vi "Load Font.vi"(11 "font directory":path) -> ()   [LabVIEW 2017]
uses:
  Default Settings.vi
panel:
  out "font overview":picture
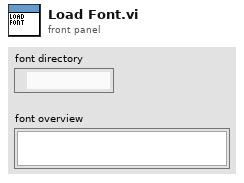
[diagram p1: front panel]
types:
  T1 = cluster{"left":i16, "top":i16, "right":i16, "bottom":i16}
  T2 = typedef "imagedata.ctl" = cluster{"image type":i32, "image depth":i32, "image":u8[], "mask":u8[], "colors":u32[], "Rectangle":cluster{"left":i16, "top":i16, "right":i16, "bottom":i16}}
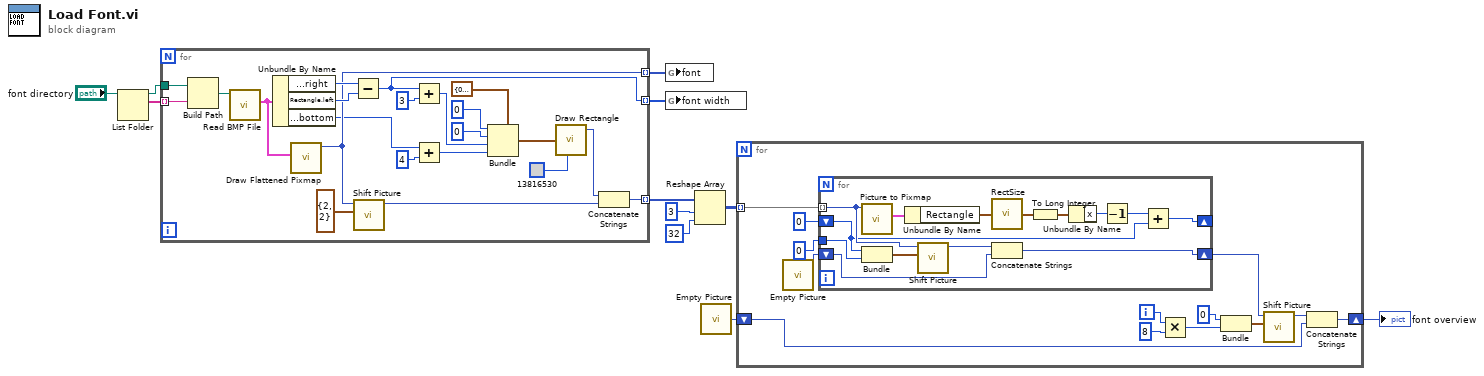
[diagram p0: block diagram]
diagram:
  n1 = List Folder(path="font directory") -> (path out=w11:path, filenames=w10:string[])  [unwired: 3 in, 2 out]
  n2 = for {
    tunnel: w10 -> [w32] mode=indexing
    tunnel: w11 -> [w33]
    tunnel: [w25] -> w8 mode=indexing
    tunnel: [w20] -> w7 mode=indexing
    tunnel: [w12] -> w6 mode=indexing
    n3 = Build Path(base path=w33, name or relative path=w32) -> (appended path=w31:path)
    n4 = call <vilib>:"Read BMP File.vi"("path to BMP file"=w31) -> ("image data"=w27:T2)  [unwired: 8 in, 2 out]
    n5 = Unbundle By Name(w27) -> ("Rectangle.right"=w30:i16, "Rectangle.left"=w29:i16, "Rectangle.bottom"=w17:i16)
    n6 = call <vilib>:"Draw Flattened Pixmap.vi"("image data"=w27) -> ("new picture"=w25:picture)  [unwired: 8 in]
    n7 = Subtract(x=w30, y=w29) -> (x-y=w20:i16)
    n8 = call "Shift Picture.vi"("shift"=cluster{"x":i16, "y":i16} {"x"=2, "y"=2}, "picture in"=w25) -> ("picture out"=w24:picture)  [unwired: 9 in]
    n9 = Add(x=w20, y=i16 3 ("x")) -> (x+y=w19:i16)
    n10 = Add(x=w17, y=i16 4) -> (x+y=w16:i16)
    n11 = Bundle(cluster=T1 {"left"=0, "top"=0, "right"=0, "bottom"=0} ("rect"), "left"=i16 0, "top"=i16 0, "right"=w19, "bottom"=w16) -> (w14:T1)
    n12 = call <vilib>:"Draw Rectangle.vi"("rect"=w14, "color(black)"=u32 13816530) -> ("new picture"=w13:picture)  [unwired: 7 in]
    n13 = Concatenate Strings(w13, w24) -> (w12:picture)
  }
  n14 = global write "Default Settings.vi" "font"(w8) -> ()
  n15 = global write "Default Settings.vi" "font width"(w7) -> ()
  n16 = Reshape Array(w6, 3 ("dimension size"), 32 ("dimension size")) -> (w3:picture[][])
  n17 = call "Empty Picture"() -> ("empty picture"=w2:picture)
  n18 = for {
    tunnel: w3 -> [w44] mode=indexing
    shift-right: [w35] -> w1
    shift-left: w2 -> [w34]
    i -> [w38]
    n19 = call "Empty Picture"() -> ("empty picture"=w45:picture)
    n20 = for {
      tunnel: w44 -> [w60] mode=indexing
      shift-right: [w50] -> _
      shift-left: 0 ("x") -> [w49]
      shift-right: [w54] -> w42
      shift-left: w45 -> [w53]
      tunnel: 0 ("x") -> [w47]
      n21 = call <vilib>:"Picture to Pixmap.vi"("picture"=w60) -> ("image data"=w59:T2)  [unwired: 9 in, 1 out]
      n22 = Bundle("x"=w49, "x"=w47) -> (w56:cluster{"x":i32, "x":i32})  [unwired: 1 in]
      n23 = Unbundle By Name(w59) -> ("Rectangle"=w58:T1)
      n24 = call "Shift Picture.vi"("shift"=w56, "picture in"=w60) -> ("picture out"=w55:picture)  [unwired: 9 in]
      n25 = call <vilib>:"RectSize.vi"("rect"=w58) -> ("point"=w57:cluster{"x":i16, "y":i16})
      n26 = Concatenate Strings(w55, w53) -> (w54:picture)
      n27 = To Long Integer(number=w57) -> (32bit integer=w48:cluster{"x":i32, "y":i32})
      n28 = Unbundle By Name(w48) -> ("x"=w52:i32)
      n29 = Decrement(x=w52) -> (x-1=w51:i32)
      n30 = Add(x=w51, y=w49) -> (x+y=w50:i32)
    }
    n31 = Multiply(x=w38, y=8 ("x")) -> (x*y=w37:i32)
    n32 = Bundle("x"=0, w37) -> (w40:cluster{"x":i32, i32})  [unwired: 1 in]
    n33 = call "Shift Picture.vi"("shift"=w40, "picture in"=w42) -> ("picture out"=w36:picture)  [unwired: 9 in]
    n34 = Concatenate Strings(w36, w34) -> (w35:picture)
  }
  "font overview" <- w1
